vi "Get Shots.vi"(11 "Series Graph in":refnum<class "Graph with Series View.lvclass">) -> (2 "Shots":u32, 3 "Series Graph out":refnum<class "Graph with Series View.lvclass">)   [LabVIEW 2025, in "Graph with Series View.lvclass"]
uses:
  Graph with Series View.lvclass
  Graph with Series View.lvclass/Graph with Series View.ctl
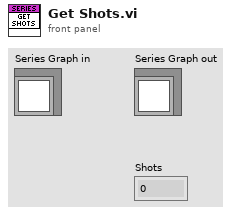
[diagram p1: front panel]
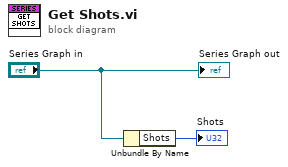
[diagram p0: block diagram]
diagram:
  n1 = Unbundle By Name("Series Graph in") -> ("Shots"=→"Shots":u32)
  "Series Graph out" <- "Series Graph in"
